vi "Fdx Convert Bytes to String Table.vi"(7 "append ASCII column?":bool, 10 "byters per row":i32=8, 11 "data":u8[](array[numeric])=[255, 255, 255, 255, 255, 255, 255, 255, 255, 255, 255, 255, 255, 255, 255, 255, 255, 255, 255, 255, 255, 255, 255, 255, 255, 255, 255, 255, 255, 255, 255, 255, 255, 255, 255, 255, 255, 255, 255, 255, 255, 255, 255, 255, 255, 255, 255, 255, 255, 255, 255, 255, 255, 255, 255, 255, 255, 255, 255, 255, 255, 255, 255, 255, 255, 255, 255, 255, 255, 255, 255, 255, 255, 255, 255, 255, 255, 255, 255, 255, 255, 255, 255, 255, 255, 255, 255, 255, 255, 255, 255, 255, 255, 255, 255, 255, 255, 255, 255, 170] format="%.0x") -> (1 "last row":u8[](array[numeric]) format="%.0x", 2 "output array":u8[][](array[numeric]) format="%.0x", 3 "data table":string[][](table))   [LabVIEW 2020, in "AIM664LV.lvlib"]
uses:
  AIM664LV.lvlib
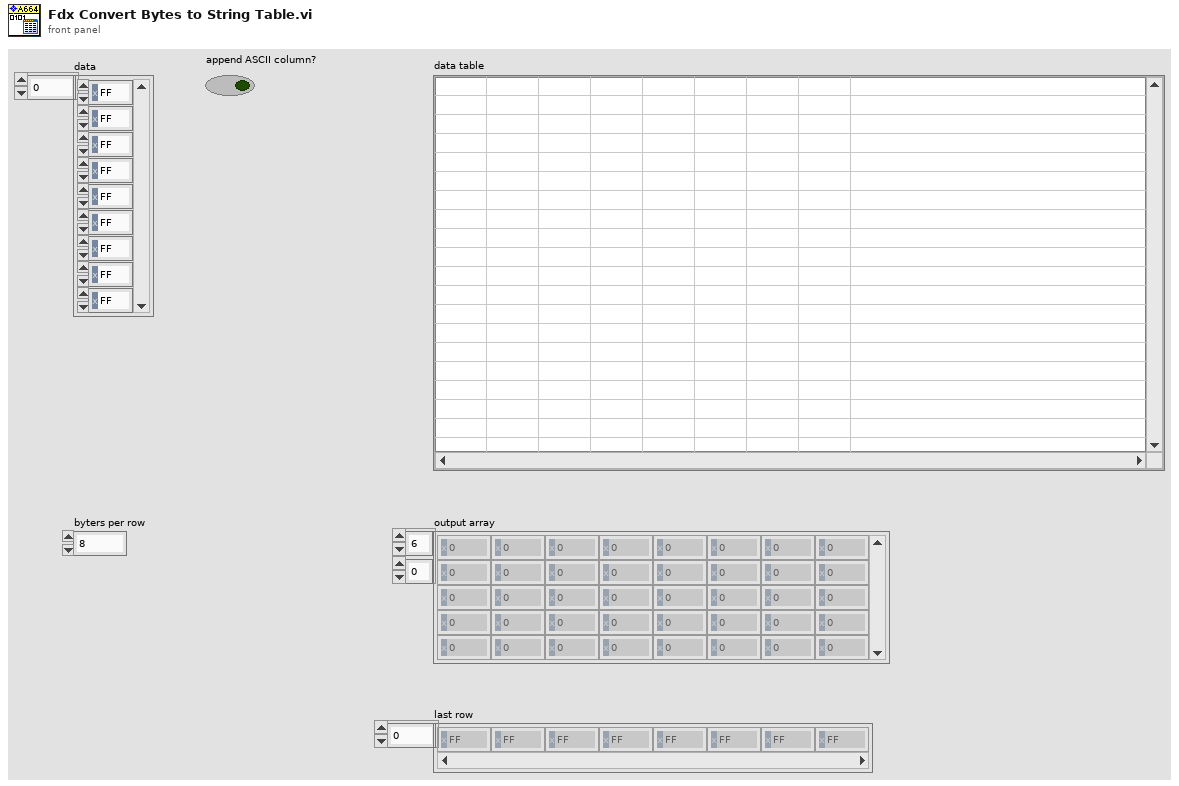
[diagram p1: front panel]
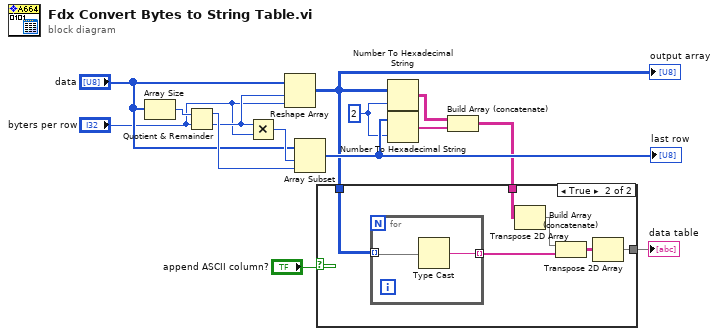
[diagram p0: block diagram]
diagram:
  w1 = i16 2 ("width (-)")
  n1 = Array Size(array="data") -> (size(s)=w14:i32)
  n2 = Quotient & Remainder(x=w14, y="byters per row") -> (x-y*floor(x/y)=w13:i32, floor(x/y)=w10:i32)
  n3 = Multiply(x=w10, y="byters per row") -> (x*y=w12:i32)
  n4 = Reshape Array("data", w10, "byters per row") -> (w5:u8[][])
  "output array" <- w5
  n5 = Array Subset(array="data", index=w12, length=w13) -> (w8:u8[])
  "last row" <- w8
  n6 = Number To Hexadecimal String(1:w1, 2:w5) -> (0:w9:string[][])
  n7 = Number To Hexadecimal String(1:w1, 2:w8) -> (0:w7:string[])
  n8 = Build Array (concatenate)(w9, w7) -> (w4:string[][])
  n9 = case shown="True" "append ASCII column?" {
    tunnel: w5 -> [_ w21]
    tunnel: w4 -> [w15 w20]
    tunnel: [w15 w17] -> w3
    frame False {
    }
    frame True {
      n10 = for {
        tunnel: w21 -> [w22] mode=indexing
        tunnel: [w23] -> w16 mode=indexing
        n11 = Type Cast(x=w22) -> (*(type *) &x=w23:string)  [unwired: 1 in]
      }
      n12 = Transpose 2D Array(2D array=w20) -> (transposed array=w18:string[][])
      n13 = Build Array (concatenate)(w18, w16) -> (w19:string[][])
      n14 = Transpose 2D Array(2D array=w19) -> (transposed array=w17:string[][])
    }
  }
  "data table" <- w3
